vi "Read Sinks.vi"(11 "Log in":refnum<class "Log.lvclass">) -> (2 "Sink DVR Array":refnum<data-value>, 3 "Log out":refnum<class "Log.lvclass">)   [LabVIEW 2019, in "TSC Event Logger.lvlib" / "Log.lvclass"]
uses:
  Log.lvclass
  Log Sinks/Log Sinks.lvclass
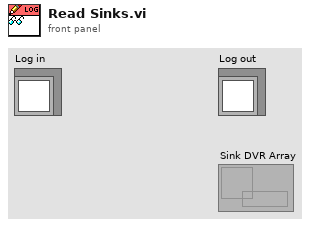
[diagram p1: front panel]
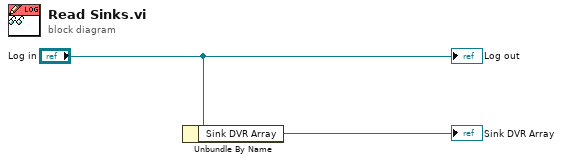
[diagram p0: block diagram]
diagram:
  n1 = Unbundle By Name("Log in") -> ("Sink DVR Array"=→"Sink DVR Array":refnum<data-value>)
  "Log out" <- "Log in"
